vi "Parse Port (Rx-UDP-CommPort).vi"(8 "error in":errorcluster, 11 "node in":refnum<k20>) -> (0 "error out":errorcluster, 3 "rx udp comm port out":T1={"PayloadID"="", "domainID"=1, "sideID"=128, "locationID"=1, "partitionID"=0, "UdpSrcPort"=0, "UdpDstPort"=0, "PortType"=enum."FDX_UDP_SAMPLING", "SubVIId"=0, "UdpNumBufMessages"=0, "UdpMaxMessageSize"=0, "UdpSamplingRate"=0, "Parameters"=[]} {"Parameters"."Parameter"."encoding" items=["BNR", "BCD", "Discrete"]})   [LabVIEW 2020, in "AIM ARINC 664 Import.lvlib"]
uses:
  AIM ARINC 664 Import.lvlib
  _typedefs/port_rx_udp_comm.ctl
  _typedefs/frame_parameter.ctl
  _typedefs/frame_parameter_definition.ctl
  Shared/Encoding (Arinc664).ctl
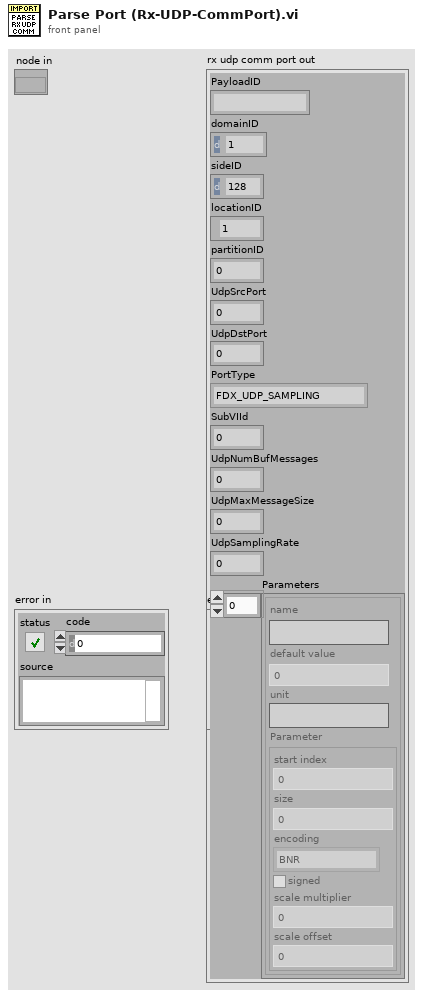
[diagram p1: front panel]
types:
  T1 = typedef "AIM ARINC 664 Import.lvlib/port_rx_udp_comm.ctl" = cluster{"PayloadID":string, "domainID":u8, "sideID":u8, "locationID":u8, "partitionID":u8, "UdpSrcPort":u16, "UdpDstPort":u16, "PortType":enum16{"FDX_UDP_SAMPLING", "FDX_UDP_QUEUING"}, "SubVIId":u32, "UdpNumBufMessages":u32, "UdpMaxMessageSize":u32, "UdpSamplingRate":u32, "Parameters":T2[]}
  T2 = typedef "AIM ARINC 664 Import.lvlib/frame_parameter.ctl" = cluster{"name":string, "default value":dbl, "unit":string, "Parameter":T3}
  T3 = typedef "AIM ARINC 664 Import.lvlib/frame_parameter_definition.ctl" = cluster{"start index":i32, "size":i32, "encoding":T4, "signed":bool, "scale multiplier":dbl, "scale offset":dbl}
  T4 = typedef "Encoding (Arinc664).ctl" = u16
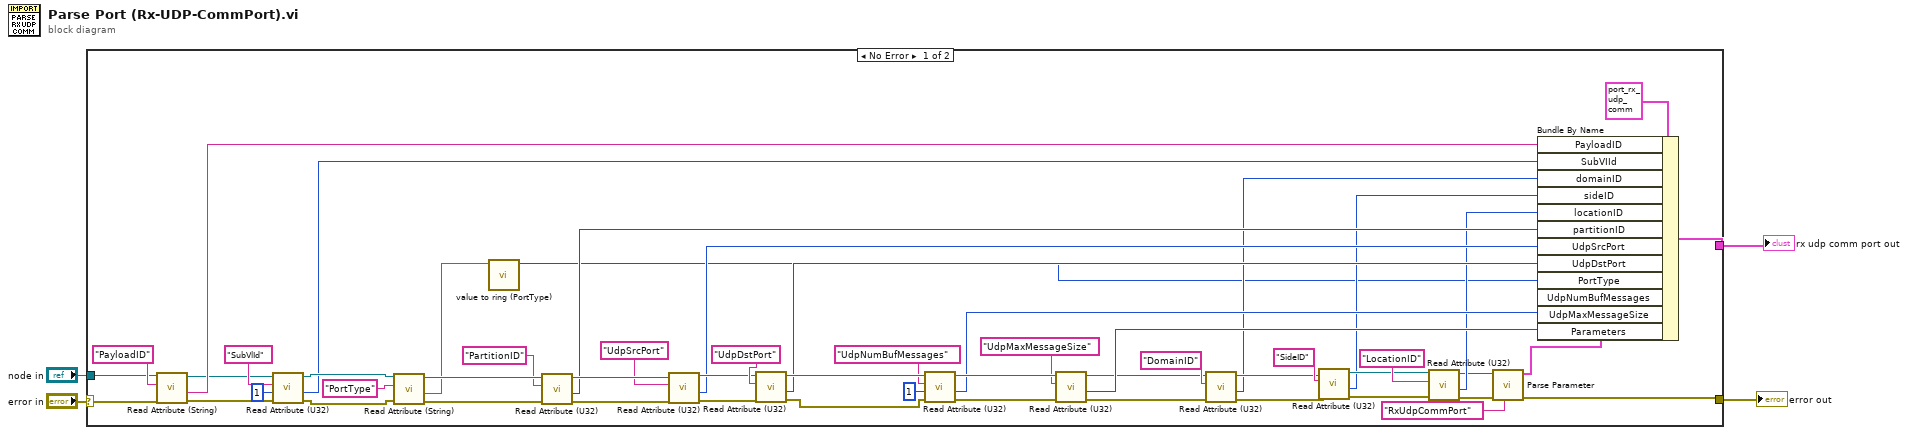
[diagram p0: block diagram]
diagram:
  n1 = case shown="No Error" "error in" {
    selector: "error in" -> [w13 w59]
    tunnel: "node in" -> [w14 _]
    tunnel: [w17 w59] -> w3
    tunnel: [w58 _] -> w1
    frame No Error {
      n2 = call "Read Attribute (String).vi"("error in"=w13, "Attribute Name"="PayloadID" ("Name"), "node in"=w14) -> ("error out"=w9:errorcluster, "value"=w12:string, "node out"=w10:refnum<k20>)  [unwired: 6 in]
      n3 = call "Read Attribute (U32).vi"("error in"=w9, "default"=u32 1, "Attribute Name"="SubVlId" ("Tag Name"), "node in"=w10) -> ("error out"=w8:errorcluster, "value"=w5:u32, "node out"=w7:refnum<k20>)  [unwired: 5 in]
      n4 = call "Read Attribute (String).vi"("error in"=w8, "Attribute Name"="PortType" ("Name"), "node in"=w7) -> ("error out"=w55:errorcluster, "value"=w23:string, "node out"=w57:refnum<k20>)  [unwired: 6 in]
      n5 = call "value to ring (PortType).vi"("value"=w23) -> ("PortType"=w22:enum16{"FDX_UDP_SAMPLING", "FDX_UDP_QUEUING"})  [unwired: 10 in]
      n6 = call "Read Attribute (U32).vi"("error in"=w55, "Attribute Name"="PartitionID" ("Tag Name"), "node in"=w57) -> ("error out"=w54:errorcluster, "value"=w36:u32, "node out"=w56:refnum<k20>)  [unwired: 6 in]
      n7 = call "Read Attribute (U32).vi"("error in"=w54, "Attribute Name"="UdpSrcPort" ("Tag Name"), "node in"=w56) -> ("error out"=w43:errorcluster, "value"=w37:u32, "node out"=w42:refnum<k20>)  [unwired: 6 in]
      n8 = call "Read Attribute (U32).vi"("error in"=w43, "Attribute Name"="UdpDstPort" ("Tag Name"), "node in"=w42) -> ("error out"=w49:errorcluster, "value"=w38:u32, "node out"=w50:refnum<k20>)  [unwired: 6 in]
      n9 = call "Read Attribute (U32).vi"("error in"=w49, "default"=u32 1, "Attribute Name"="UdpNumBufMessages" ("Tag Name"), "node in"=w50) -> ("error out"=w48:errorcluster, "value"=w39:u32, "node out"=w47:refnum<k20>)  [unwired: 5 in]
      n10 = call "Read Attribute (U32).vi"("error in"=w48, "Attribute Name"="UdpMaxMessageSize" ("Tag Name"), "node in"=w47) -> ("error out"=w34:errorcluster, "value"=w40:u32, "node out"=w32:refnum<k20>)  [unwired: 6 in]
      n11 = call "Read Attribute (U32).vi"("error in"=w34, "Attribute Name"="DomainID" ("Tag Name"), "node in"=w32) -> ("error out"=w31:errorcluster, "value"=w24:u32, "node out"=w28:refnum<k20>)  [unwired: 6 in]
      n12 = call "Read Attribute (U32).vi"("error in"=w31, "Attribute Name"="SideID" ("Tag Name"), "node in"=w28) -> ("error out"=w30:errorcluster, "value"=w25:u32, "node out"=w27:refnum<k20>)  [unwired: 6 in]
      n13 = call "Read Attribute (U32).vi"("error in"=w30, "Attribute Name"="LocationID" ("Tag Name"), "node in"=w27) -> ("error out"=w19:errorcluster, "value"=w26:u32, "node out"=w20:refnum<k20>)  [unwired: 6 in]
      n14 = call "Parse Parameter.vi"("error text in"="RxUdpCommPort", "error in"=w19, "node in"=w20) -> ("error out"=w17:errorcluster, "parametesrs"=w18:T2[])  [unwired: 7 in]
      n15 = Bundle By Name(cluster=T1 {"PayloadID"="", "domainID"=1, "sideID"=128, "locationID"=1, "partitionID"=0, "UdpSrcPort"=0, "UdpDstPort"=0, "PortType"=enum."FDX_UDP_SAMPLING", "SubVIId"=0, "UdpNumBufMessages"=0, "UdpMaxMessageSize"=0, "UdpSamplingRate"=0, "Parameters"=[]} ("session_tx_generic"), "PayloadID"=w12, "SubVIId"=w5, "domainID"=w24, "sideID"=w25, "locationID"=w26, "partitionID"=w36, "UdpSrcPort"=w37, "UdpDstPort"=w38, "PortType"=w22, "UdpNumBufMessages"=w39, "UdpMaxMessageSize"=w40, "Parameters"=w18) -> (w58:T1)
    }
    frame Error {
    }
  }
  "error out" <- w3
  "rx udp comm port out" <- w1
